vi "Set FlatSequence Subdiagram Label.vi"(8 "error in (no error)":errorcluster, 9 "QD Combo Box Ref":refnum<vi>, 10 "Shift Not Pressed?":bool, 11 "FlatSequence in":refnum<vi>) -> (0 "error out":errorcluster)   [LabVIEW 2017]
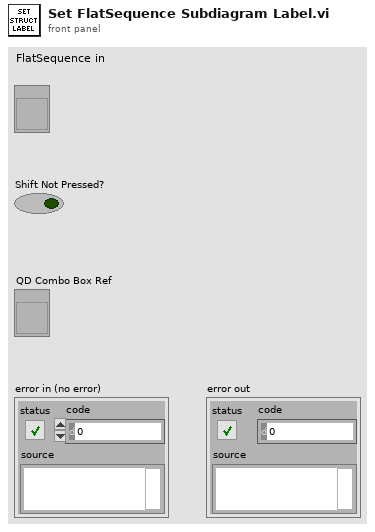
[diagram p1: front panel]
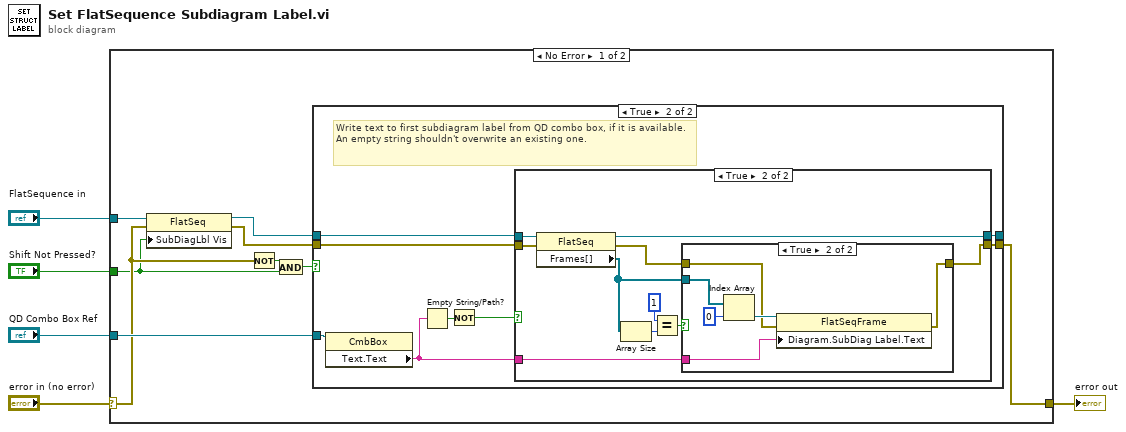
[diagram p0: block diagram]
diagram:
  n1 = case shown="No Error" "error in (no error)" {
    selector: "error in (no error)" -> [w7 w44]
    tunnel: [w11 w44] -> w5
    tunnel: "Shift Not Pressed?" -> [w6 _]
    tunnel: "QD Combo Box Ref" -> [w14 _]
    tunnel: "FlatSequence in" -> [w10 _]
    frame No Error {
      n2 = property class="FlatSeq"(reference=w10, error in=w7, "SubDiagLbl Vis"=w6) -> (reference out=w9:refnum<vi>, error out=w8:errorcluster)
      n3 = Not(x=w7) -> (.not. x?=w13:bool)
      n4 = And(x=w13, y=w6) -> (x .and. y?=w12:bool)
      n5 = case shown="True" w12 {
        tunnel: w14 -> [_ w24]
        tunnel: w9 -> [w16 w17]
        tunnel: [w16 w23] -> _
        tunnel: [w15 w22] -> w11
        tunnel: w8 -> [w15 w18]
        frame False {
        }
        frame True {
          # "Write text to first subdiagram label from QD combo box, if it is available. An empty string shouldn't overwrite an existing one."
          n6 = property class="CmbBox"(reference=w24) -> ("Text.Text"=w21:string)  [unwired: 1 in, 2 out]
          n7 = Empty String/Path?(string/path=w21) -> (empty?=w19:bool)
          n8 = Not(x=w19) -> (.not. x?=w20:bool)
          n9 = case shown="True" w20 {
            tunnel: [w26 w28] -> w23
            tunnel: [w25 w36] -> w22
            tunnel: w18 -> [w25 w35]
            tunnel: w17 -> [w26 w32]
            tunnel: w21 -> [_ w34]
            frame False {
            }
            frame True {
              n10 = property class="FlatSeq"(reference=w32, error in=w35) -> (reference out=w28:refnum<vi>, error out=w33:errorcluster, "Frames[]"=w29:refnum<vi>[])
              n11 = Array Size(array=w29) -> (size(s)=w31:i32)
              n12 = Equal?(x=1, y=w31) -> (x = y?=w30:bool)
              n13 = case shown="True" w30 {
                tunnel: [w37 w39] -> w36
                tunnel: w34 -> [_ w41]
                tunnel: w33 -> [w37 w40]
                tunnel: w29 -> [_ w38]
                frame False {
                }
                frame True {
                  n14 = Index Array(array=w38, index=0) -> (element=w42:refnum<vi>)
                  n15 = property class="FlatSeqFrame"(reference=w42, error in=w40, "Diagram.SubDiag Label.Text"=w41) -> (error out=w39:errorcluster)  [unwired: 1 out]
                }
              }
            }
          }
        }
      }
    }
    frame Error {
    }
  }
  "error out" <- w5
